vi "Coins.vi"(8 "error in (no error)":errorcluster, 10 "Coins":T1, 11 "Monedas USD in":refnum<class "Monedas USD.lvclass">) -> (0 "error out":errorcluster, 3 "Monedas USD out":refnum<class "Monedas USD.lvclass">)   [LabVIEW 2020, in "Monedas USD.lvlib" / "Monedas USD.lvclass"]
uses:
  Monedas USD.lvclass
  C:/Program Files (x86)/National Instruments/LabVIEW 2020/vi.lib/ActorFramework/Actor/Actor.lvclass
  <vilib>/ActorFramework/Actor/Actor.lvclass/Actor.ctl
  Monedas USD.lvclass/Monedas USD.ctl
  UI Actor Messages/Add credit Msg/Add credit Msg.lvclass/Add credit Msg.ctl
  <vilib>/ActorFramework/Message Enqueuer/Message Enqueuer.lvclass/Message Enqueuer.ctl
  <vilib>/ActorFramework/Message Enqueuer/Enqueue.vi
  UI Actor Messages/Add credit Msg/Add credit Msg.lvclass
  C:/Program Files (x86)/National Instruments/LabVIEW 2020/vi.lib/ActorFramework/Message/Message.lvclass
  <vilib>/ActorFramework/Message Priority Queue/Priority Enqueue.vi
  <vilib>/ActorFramework/Actor/Actor.lvclass
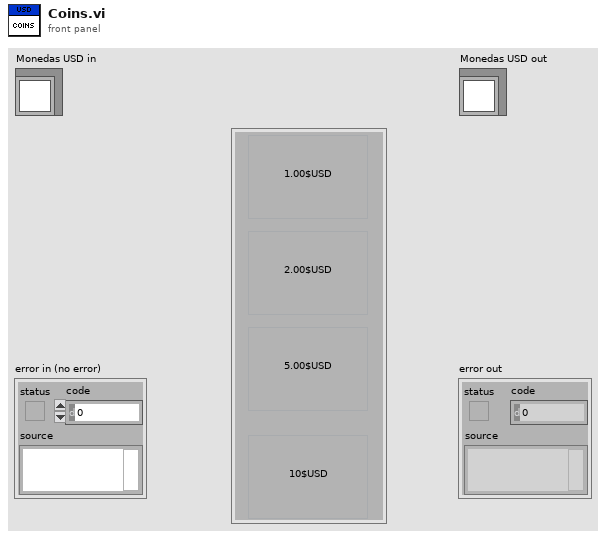
[diagram p1: front panel]
types:
  T1 = cluster{"1 2":bool, "2 2":bool, "5 3":bool, "5 4":bool}
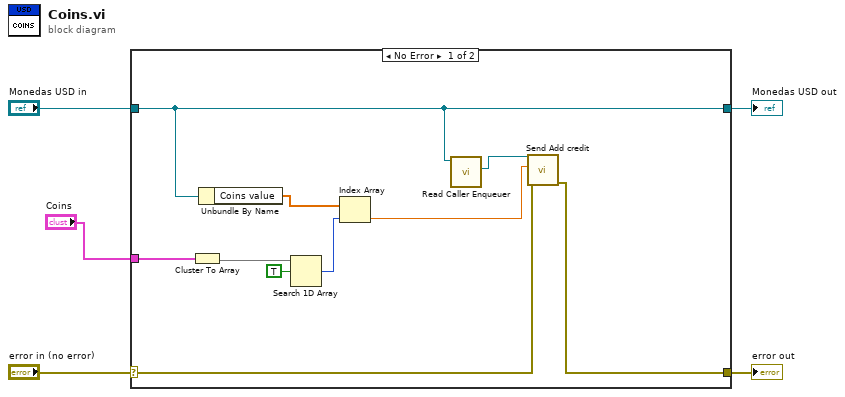
[diagram p0: block diagram]
diagram:
  n1 = case shown="No Error" "error in (no error)" {
    selector: "error in (no error)" -> [w8 w17]
    tunnel: [w7 w17] -> w4
    tunnel: [w10 w16] -> w2
    tunnel: "Monedas USD in" -> [w10 w16]
    tunnel: "Coins" -> [w9 _]
    frame No Error {
      n2 = Cluster To Array(cluster=w9) -> (array=w15:bool[])
      n3 = Unbundle By Name(w10) -> ("Coins value"=w12:dbl[])
      n4 = Search 1D Array(1D array=w15, element=TRUE) -> (index of element=w14:i32)  [unwired: 1 in]
      n5 = Index Array(array=w12, index=w14) -> (element=w11:dbl)
      n6 = call <vilib>:"Read Caller Enqueuer.vi"("Actor"=w10) -> ("Caller Enqueuer"=w13:refnum<class "Message Enqueuer.lvclass">)  [unwired: 10 in]
      n7 = call "Send Add credit.vi"("error in (no error)"=w8, "Credito"=w11, "Message Enqueuer"=w13) -> ("error out"=w7:errorcluster)  [unwired: 7 in, 1 out]
    }
    frame Error {
    }
  }
  "error out" <- w4
  "Monedas USD out" <- w2
